vi "Function.vi"(8 "error in (no error)":errorcluster, 9 "Numeric":dbl, 10 "Waveform":waveform(dbl), 11 "Two Terminal in":refnum<class "Divide_WFM_Numeric.lvclass">) -> (0 "error out":errorcluster, 2 "Result":waveform(dbl), 3 "Two Terminal out":refnum<class "Divide_WFM_Numeric.lvclass">)   [LabVIEW 2021, in "Divide_WFM_Numeric.lvclass"]
uses:
  Divide_WFM_Numeric.lvclass
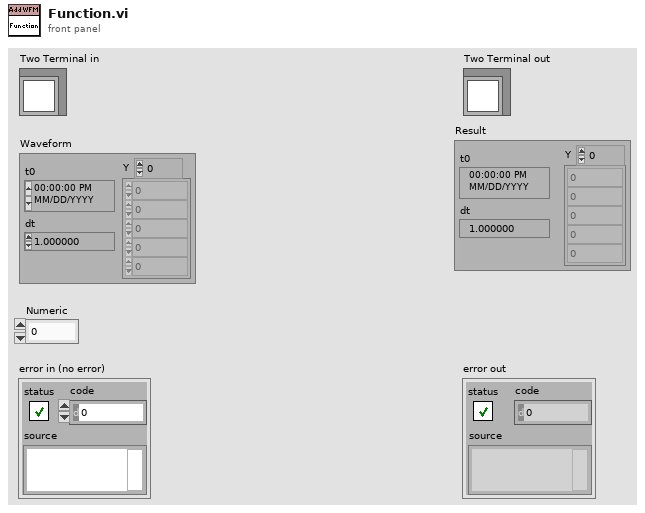
[diagram p1: front panel]
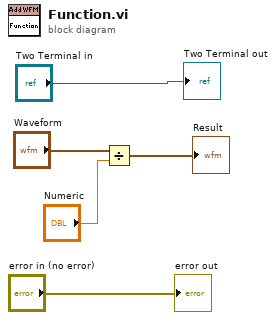
[diagram p0: block diagram]
diagram:
  n1 = Divide(x="Waveform", y="Numeric") -> (x/y=→"Result":waveform(dbl))
  "error out" <- "error in (no error)"
  "Two Terminal out" <- "Two Terminal in"
